vi "Vehicle Status to RIO OK.vi"(10 "Vehicle Status":T1) -> (2 "RIO OK":bool)   [LabVIEW 2014]
uses:
  Vehicle Status/Subsystem Status.ctl
  Vehicle Status/Subsystem Status Severity.ctl
  Vehicle Status/Subsystem Status Message.ctl
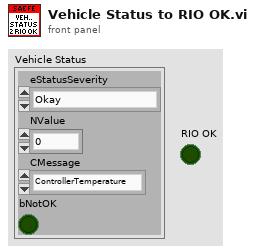
[diagram p1: front panel]
types:
  T1 = typedef "Subsystem Status.ctl" = cluster{"eStatusSeverity":T2, "NValue":sgl, "CMessage":T3, "bNotOK":bool}
  T2 = typedef "Subsystem Status Severity.ctl" = enum16{"Okay", "Short Warning", "Long Warning", "Return to Pits", "Error", "Danger"}
  T3 = typedef "Subsystem Status Message.ctl" = enum16{"ControllerTemperature", "MotorTemperature", "BatteryTemperature", "BatteryLowVoltage", "LVBattery", "sbRIOTemperature", "Precharge", "BSPD", "IMD", "RemoteReturnToPits", "EStopInterrupted", "NoCellComms", "MCOverSpeed", "MCOverCurrent", "MCOverVoltage", "MCInverterOverTemp", "MCDirectionCommand", "MCInverterTimeout", "MCDesatFault", "MCHWOverCurrent", "MCUnderVoltage", "MCCommandMessageLost", "MotorOverTemp", "MCModAOverTemp", "MCModBOverTemp", "MCModCOverTemp", "MCPCBOverTemp", "MCGateDrv1OverTemp", "MCDateDrv2OverTemp", "MCCurrentSensorFault", "MCResolverNotConnected", "ShutdownLatchTripped", "UnknownBMS", "RemoteEmergency"}
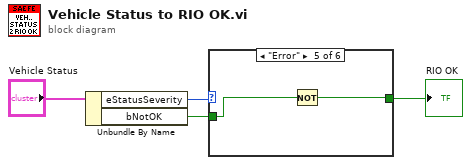
[diagram p0: block diagram]
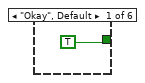
[diagram p2: hidden frame]
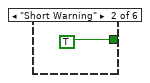
[diagram p3: hidden frame]
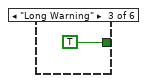
[diagram p4: hidden frame]
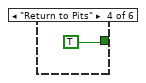
[diagram p5: hidden frame]
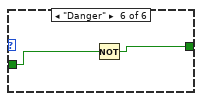
[diagram p6: hidden frame]
diagram:
  n1 = Unbundle By Name("Vehicle Status") -> ("eStatusSeverity"=w2:T2, "bNotOK"=w1:bool)
  n2 = case shown="\"Error\"" w2 {
    tunnel: [TRUE ("RIO OK") TRUE ("RIO OK") TRUE ("RIO OK") TRUE ("RIO OK") w9 w11] -> w4
    tunnel: w1 -> [_ _ _ _ w10 w12]
    frame "Okay", Default {
    }
    frame "Short Warning" {
    }
    frame "Long Warning" {
    }
    frame "Return to Pits" {
    }
    frame "Error" {
      n3 = Not(x=w10) -> (.not. x?=w9:bool)
    }
    frame "Danger" {
      n4 = Not(x=w12) -> (.not. x?=w11:bool)
    }
  }
  "RIO OK" <- w4
